vi "Set Gantry Head Vacuum.vi"(7 "Gantry Class in":refnum<class "Gantry Class.lvclass">, 8 "error in (no error)":errorcluster, 9 "On/Off":bool, 10 "Inner/Outer":enum16{"Outer", "Inner"}(ring)) -> (0 "error out":errorcluster, 5 "Gantry Class out":refnum<class "Gantry Class.lvclass">)   [LabVIEW 2011, in "Gantry Class.lvclass"]
uses:
  Gantry Class.lvclass
  WorkTable Class/WorkTable Class.lvclass
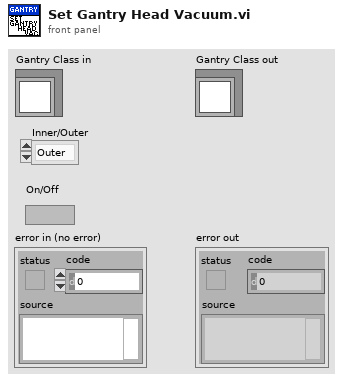
[diagram p1: front panel]
types:
  T1 = typedef "Worktable_Gantry Head.ctl" = cluster{"Current Tool":enum16{"None", "Grabber", "Picker", "Tool Setter"}, "Vacuum Channel Inner":u8, "Vacuum Channel Outer":u8}
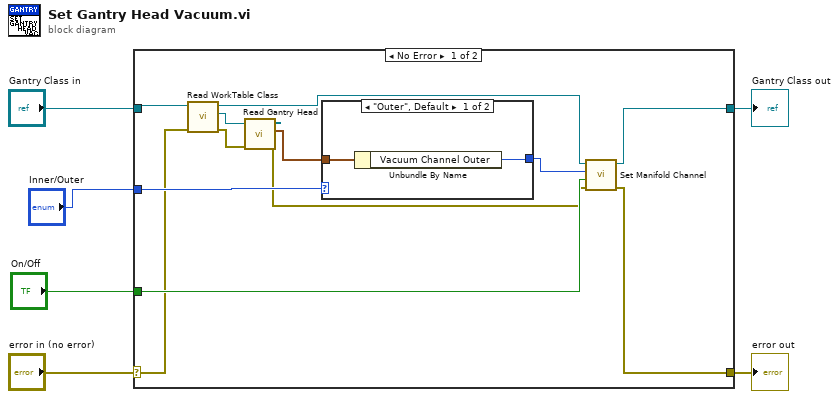
[diagram p0: block diagram]
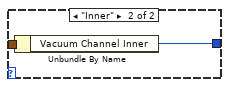
[diagram p2: hidden frame]
diagram:
  n1 = case shown="No Error" "error in (no error)" {
    selector: "error in (no error)" -> [w8 w24]
    tunnel: [w7 w24] -> w5
    tunnel: [w11 w23] -> w3
    tunnel: "Gantry Class in" -> [w18 w23]
    tunnel: "Inner/Outer" -> [w16 _]
    tunnel: "On/Off" -> [w14 _]
    frame No Error {
      n2 = call "Read WorkTable Class.vi"("error in (no error)"=w8, "Gantry Class in"=w18) -> ("error out"=w10:errorcluster, "WorkTable Class.lvclass"=w17:refnum<class "WorkTable Class.lvclass">, "Gantry Class out"=w12:refnum<class "Gantry Class.lvclass">)  [unwired: 7 in]
      n3 = call-dynamic "Read Gantry Head.vi"("error in (no error)"=w10, "WorkTable Class in"=w17) -> ("error out"=w9:errorcluster, "Gantry Head"=w15:T1)  [unwired: 7 in, 1 out]
      n4 = case shown="\"Outer\", Default" w16 {
        tunnel: w15 -> [w20 w22]
        tunnel: [w19 w21] -> w13
        frame "Outer", Default {
          n5 = Unbundle By Name(w20) -> ("Vacuum Channel Outer"=w19:u8)
        }
        frame "Inner" {
          n6 = Unbundle By Name(w22) -> ("Vacuum Channel Inner"=w21:u8)
        }
      }
      n7 = call "Set Manifold Channel.vi"("error in (no error)"=w9, "On/Off"=w14, "Manifold Channel"=w13, "Gantry Class in"=w12) -> ("error out"=w7:errorcluster, "Gantry Class out"=w11:refnum<class "Gantry Class.lvclass">)  [unwired: 6 in]
    }
    frame Error {
    }
  }
  "error out" <- w5
  "Gantry Class out" <- w3
